vi "AuslesenVonKalibrierung.vi"(7 "Error in":errorcluster, 10 "EMTestCWS500N.lvclass":refnum<class "EMTestCWS500N.lvclass">) -> (0 "error out":errorcluster, 1 "output":string, 3 "EMTestCWS500N out":refnum<class "EMTestCWS500N.lvclass">)   [LabVIEW 2013, in "EMTestCWS500N.lvclass"]
uses:
  EMTestCWS500N.lvclass
  Main/controls/TestData.ctl
  Main/controls/TestStates.ctl
  lib/EMV-Test.lvlib
panel:
  out "Fortschritt":dbl(slide) scale=0.0..1.0
  out "String":string
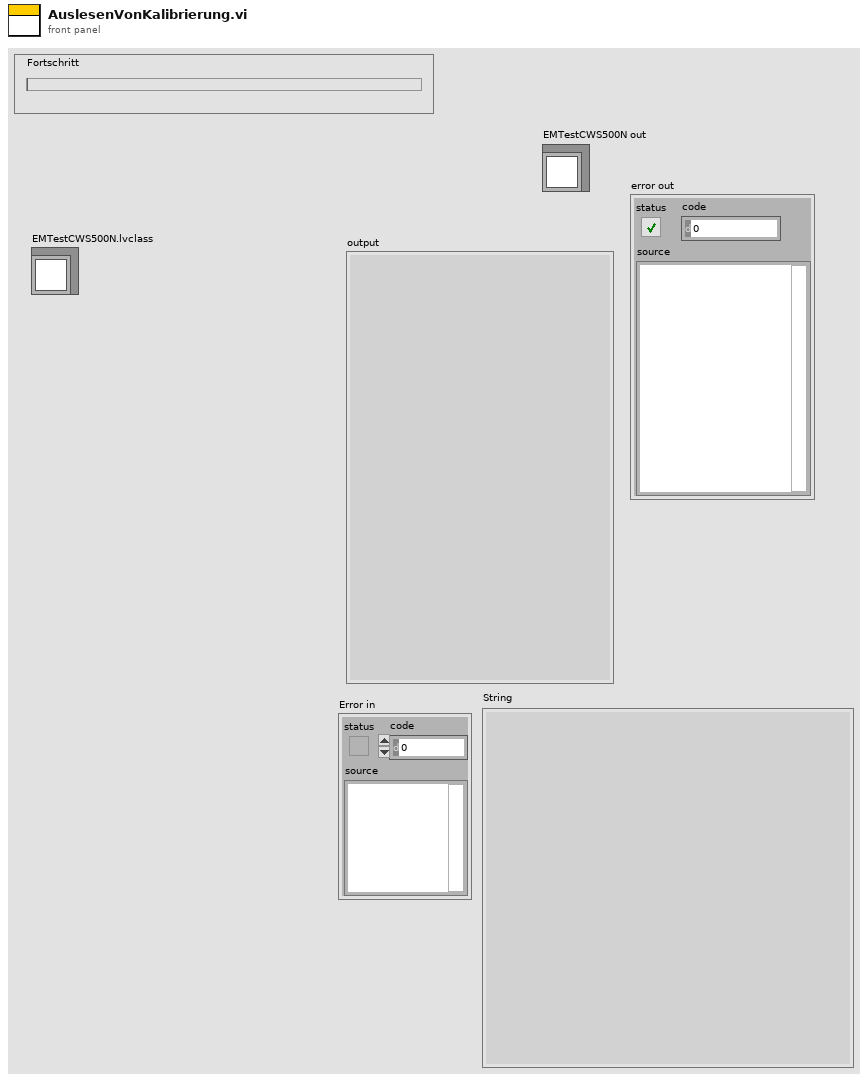
[diagram p1: front panel]
types:
  T1 = typedef "EMV-Test.lvlib/TestData.ctl" = cluster{"commandlist":string, "line":i32, "last response":string, "timeout":i32, "wait":u32, "erfolgreich":bool, "next state":T2}
  T2 = typedef "EMV-Test.lvlib/TestStates.ctl" = enum16{"check for pressed Buttons", "pause", "vorgefertigter Test", "manueller Test", "respond to response", "error", "Start", "Initialise", "open connection", "evaluate line", "wait for Response", "wait", "catch error", "close Connection", "end", "empty buffer"}
  T3 = enum16{"open", "replace", "create", "open or create", "replace or create", "replace or create with confirmation"}
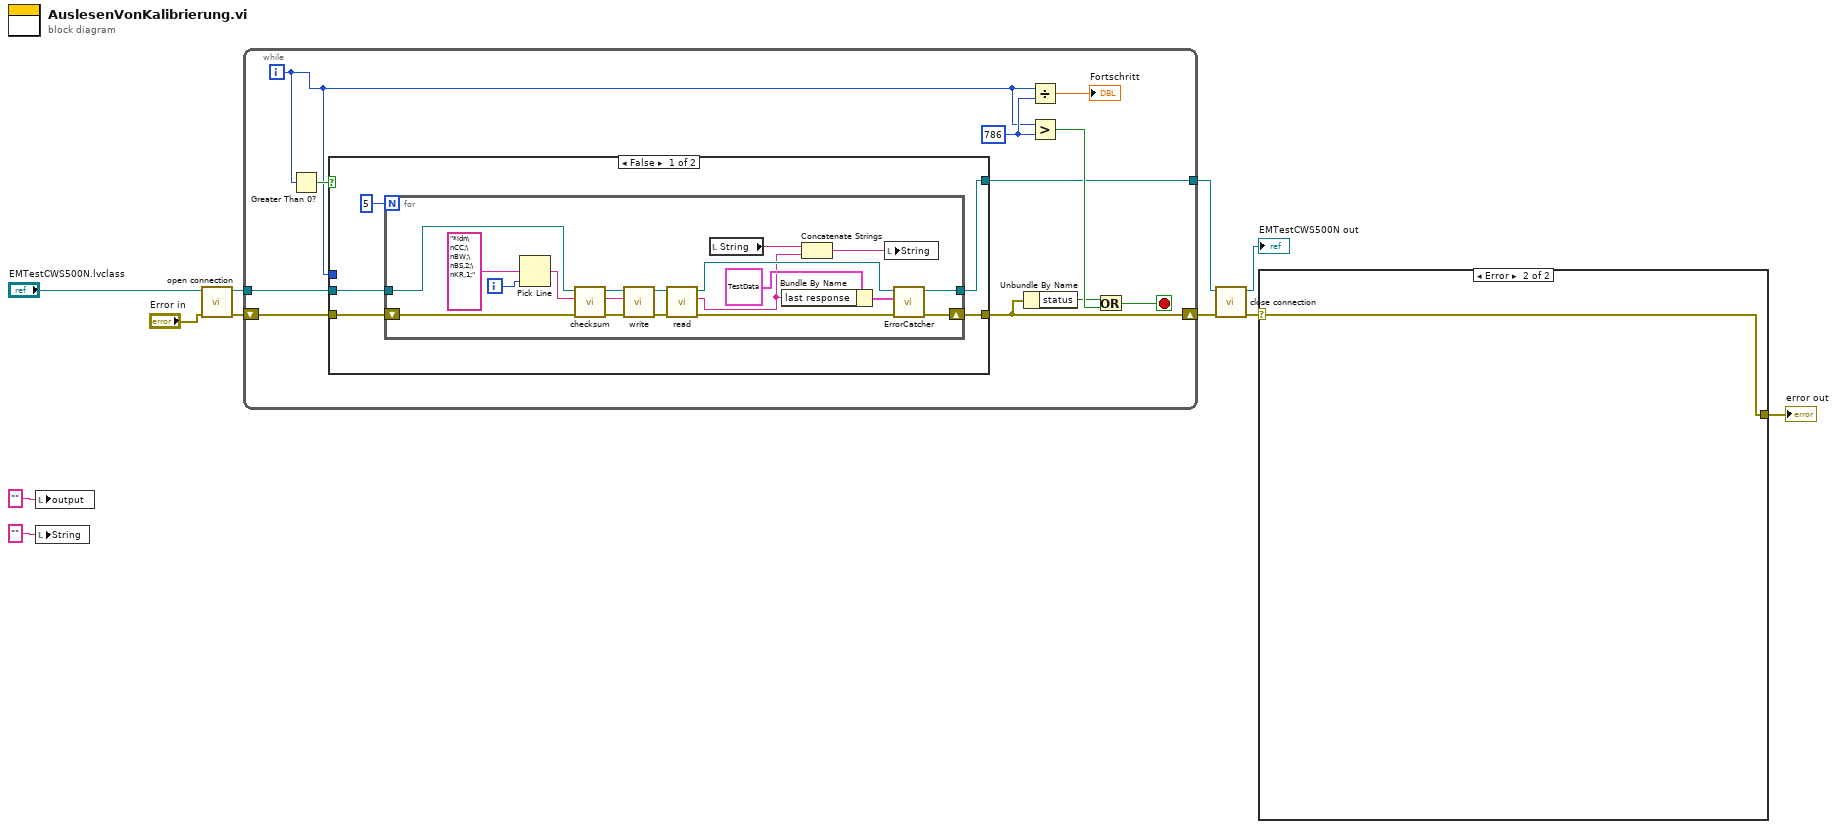
[diagram p0: block diagram]
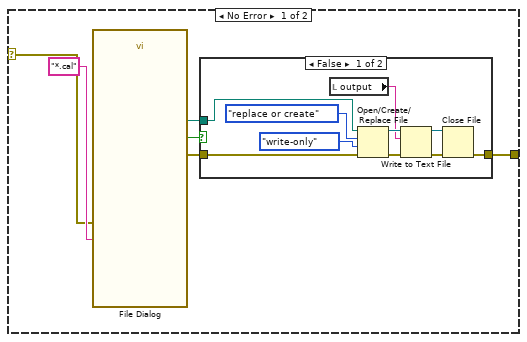
[diagram p2: hidden frame]
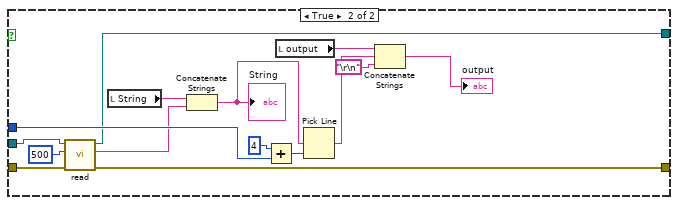
[diagram p4: hidden frame]
diagram:
  n1 = local write "output"("") -> ()
  n2 = local write "String"("") -> ()
  n3 = call-dynamic "open connection.vi"("error in (no error)"="Error in", "EMTestCWS500N in"="EMTestCWS500N.lvclass") -> ("error out"=w9:errorcluster, "EMTestCWS500N out"=w8:refnum<class "EMTestCWS500N.lvclass">)  [unwired: 8 in]
  n4 = while {
    shift-right: [w19] -> w10
    shift-left: w9 -> [w15]
    tunnel: [w17] -> w11
    tunnel: w8 -> [w16]
    i -> [w12]
    stop <- w20 stop-if-true
    w13 = 786 ("y")
    n5 = Greater Than 0?(x=w12) -> (x > 0?=w22:bool)
    n6 = case shown="False" w22 {
      tunnel: [w27 w50] -> w19
      tunnel: w12 -> [_ w58]
      tunnel: [w23 w49] -> w17
      tunnel: w16 -> [w24 w47]
      tunnel: w15 -> [w25 w48]
      frame False {
        n7 = for {
          N: 5 -> [_]
          shift-right: [w31] -> w27
          shift-left: w25 -> [w35]
          tunnel: w24 -> [w34]
          tunnel: [w32] -> w23
          i -> [w46]
          n8 = Pick Line(multi-line string="*idn\nCC;\nBW;\nBS,2;\nKR,1;", line index=w46) -> (output string=w40:string)  [unwired: 1 in]
          n9 = call-dynamic "checksum.vi"("error in (no error)"=w35, "input"=w40, "EMTestCWS500N in"=w34) -> ("error out"=w41:errorcluster, "output"=w33:string, "EMTestCWS500N out"=w42:refnum<class "EMTestCWS500N.lvclass">)  [unwired: 6 in]
          n10 = call-dynamic "write.vi"("error in (no error)"=w41, "String to send"=w33, "EMTestCWS500N in"=w42) -> ("error out"=w38:errorcluster, "EMTestCWS500N out"=w39:refnum<class "EMTestCWS500N.lvclass">)  [unwired: 7 in]
          n11 = call-dynamic "read.vi"("error in (no error)"=w38, "EMTestCWS500N in"=w39) -> ("error out"=w37:errorcluster, "Return String"=w29:string, "EMTestCWS500N out"=w36:refnum<class "EMTestCWS500N.lvclass">)  [unwired: 7 in]
          n12 = local read "String"() -> (w43:string)
          n13 = Bundle By Name(cluster=T1 {"commandlist"="", "line"=0, "last response"="", "timeout"=0, "wait"=0, "erfolgreich"=FALSE, "next state"=enum."check for pressed Buttons"}, "last response"=w29) -> (w28:T1)
          n14 = Concatenate Strings(w43, w29) -> (w44:string)
          n15 = local write "String"(w44) -> ()
          n16 = call-dynamic "ErrorCatcher.vi"("error in (no error)"=w37, 10:w28, "EMTestCWS500N in"=w36) -> ("error out"=w31:errorcluster, "EMTestCWS500N out"=w32:refnum<class "EMTestCWS500N.lvclass">)  [unwired: 7 in]
        }
      }
      frame True {
        n17 = call-dynamic "read.vi"("error in (no error)"=w48, "timeout (ms)"=500, "EMTestCWS500N in"=w47) -> ("error out"=w50:errorcluster, "Return String"=w51:string, "EMTestCWS500N out"=w49:refnum<class "EMTestCWS500N.lvclass">)  [unwired: 6 in]
        n18 = local read "String"() -> (w61:string)
        n19 = Concatenate Strings(w61, w51) -> (w54:string)
        "String" <- w54
        n20 = Add(x=u32 4, y=w58) -> (x+y=w60:u32)
        n21 = local read "output"() -> (w56:string)
        n22 = Pick Line(multi-line string=w54, line index=w60) -> (output string=w57:string)  [unwired: 1 in]
        n23 = Concatenate Strings(w56, w57, "\r\n") -> (→"output":string)
      }
    }
    n24 = Unbundle By Name(w19) -> ("status"=w18:bool)
    n25 = Divide(x=w12, y=w13) -> (x/y=→"Fortschritt":dbl)
    n26 = Greater?(x=w12, y=w13) -> (0:w21:bool)
    n27 = Or(x=w18, y=w21) -> (x .or. y?=w20:bool)
  }
  n28 = call-dynamic "close connection.vi"("error in (no error)"=w10, "EMTestCWS500N in"=w11) -> ("error out"=w7:errorcluster, "EMTestCWS500N out"=→"EMTestCWS500N out":refnum<class "EMTestCWS500N.lvclass">)  [unwired: 8 in]
  n29 = case shown="Error" w7 {
    selector: w7 -> [w65 w79]
    tunnel: [w62 w79] -> w6
    frame No Error {
      n30 = call "File Dialog"("error in"=w65, "pattern (all files)"="*.cal") -> ("selected path"=w64:path, "cancelled"=w63:bool, "error out"=w66:errorcluster)  [unwired: 10 in, 1 out]
      n31 = case shown="False" w63 {
        tunnel: w66 -> [w77 w78]
        tunnel: w64 -> [w71 _]
        tunnel: [w69 w78] -> w62
        frame False {
          n32 = local read "output"() -> (w72:string)
          n33 = Open/Create/Replace File(file path (use dialog)=w71, error in=w77, operation (0:open)=T3."replace or create", access (0:read/write)=enum16{"read/write", "read-only", "write-only"}."write-only") -> (refnum out=w76:refnum<file>, error out=w75:errorcluster)  [unwired: 2 in, 1 out]
          n34 = Write to Text File(file (use dialog)=w76, text=w72, error in=w75) -> (refnum out=w73:refnum<file>, error out=w74:errorcluster)  [unwired: 1 in, 1 out]
          n35 = Close File(refnum=w73, error in=w74) -> (error out=w69:errorcluster)  [unwired: 1 out]
        }
        frame True {
        }
      }
    }
    frame Error {
    }
  }
  "error out" <- w6
